vi "main.vi"() -> ()   [LabVIEW 2014]
uses:
  <vilib>/Instr/_visa.llb/VISA Configure Serial Port (Instr).vi
  <vilib>/picture/3D Picture Control/Object/Create Object (name).vi
  <vilib>/picture/3D Picture Control/NI_3D Picture Control.lvlib
panel:
  out "CALIB GZ":dbl
  out "CALIB GY":dbl
  out "CALIB GX":dbl
  out "RAW GZ":string
  out "RAW GY":string
  out "RAW GX":string
  out "ACCELEROMETER":T1(graph)
  out "AZ":string
  out "AY":string
  out "Simulator":refnum<vi>(3d-picture)
  out "CALIB GYROMETER":T1(graph)
  in  "stop":bool
  out "BYTE COUNT:":dbl
  in  "COM Port":refnum<visa-resource-name>
  out "AX":string
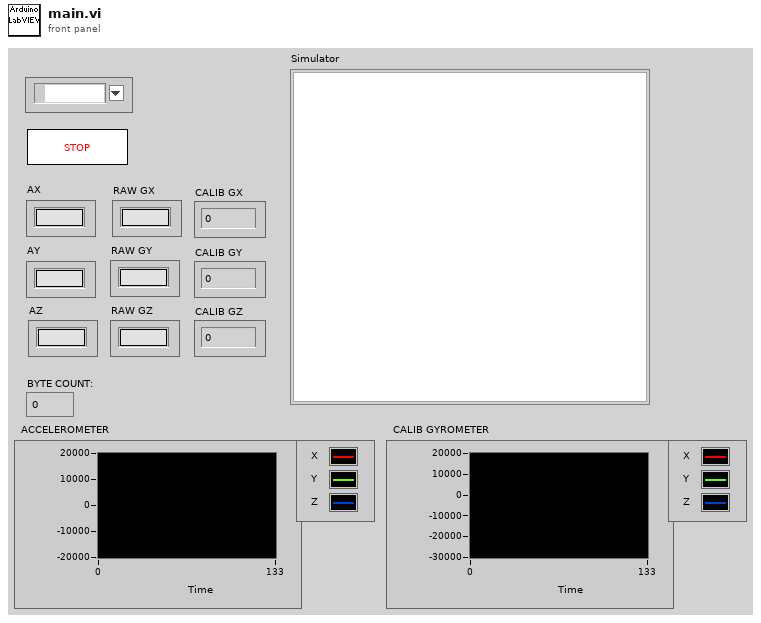
[diagram p1: front panel]
types:
  T1 = cluster{"read buffer":i32, "trimmed string":i32, "trimmed string":i32}
  T2 = enum16{"As a Decal", "With Modulation", "With Blending", "As a replacement"}
  T3 = cluster{"Red":sgl, "Green":sgl, "Blue":sgl, "Alpha":sgl}
  T4 = typedef "imagedata.ctl" = cluster{"image type":i32, "image depth":i32, "image":u8[], "mask":u8[], "colors":u32[], "Rectangle":cluster{"left":i16, "top":i16, "right":i16, "bottom":i16}}
  T5 = cluster{"trimmed string":string, "trimmed string":string, "trimmed string":string}
  T6 = cluster{"trimmed string":i32, "trimmed string":i32, "trimmed string":i32}
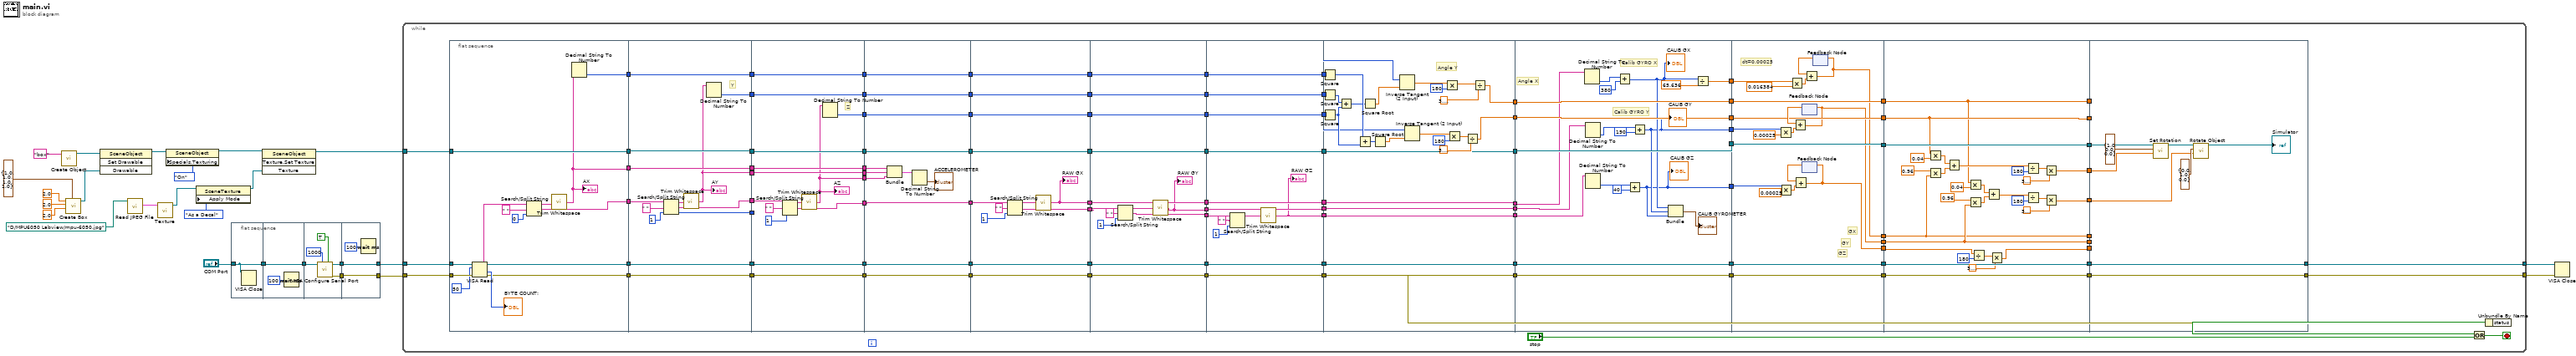
[diagram p0: block diagram]
diagram:
  n1 = call-poly <vilib>:"Create Object.vi"("Name"="box") -> ("Scene:New Object"=w1:refnum<vi>)  [unwired: 9 in, 1 out]
  n2 = call <vilib>:"Create Box.vi"("Color"=T3 {"Red"=1.0, "Green"=1.0, "Blue"=1.0, "Alpha"=1.0}, "Length Z"=2.0, "Length Y"=2.0, "Length X"=2.0) -> ("New Box Refnum"=w12:refnum<vi>)  [unwired: 6 in, 1 out]
  n3 = invoke class="SceneObject" method="Set Drawable"(reference=w1, "Drawable"=w12) -> (reference out=w2:refnum<vi>)  [unwired: 2 in, 3 out]
  n4 = call <vilib>:"Read JPEG File.vi"("path to JPEG file"=path "D:/MPU6050 Labview/mpu-6050.jpg") -> ("image data"=w11:T4)  [unwired: 8 in, 2 out]
  n5 = call <vilib>:"Texture.vi"("Image"=w11) -> ("New Texture Refnum"=w9:refnum<vi>)  [unwired: 9 in, 1 out]
  n6 = property class="SceneObject"(reference=w2, "Specials.Texturing"=enum16{"Inherit Value", "Off", "On"}."On" ("Specials:Texturing")) -> (reference out=w4:refnum<vi>)  [unwired: 1 in, 1 out]
  n7 = property class="SceneTexture"(reference=w9, "Apply Mode"=T2."As a Decal") -> (reference out=w10:refnum<vi>)  [unwired: 1 in, 1 out]
  n8 = flat-sequence {
    tunnel: "COM Port" -> [w26]
    tunnel: [w26] -> w25
    tunnel: w25 -> [w28]
    tunnel: [w28] -> w24
    tunnel: w24 -> [w33]
    tunnel: [w32] -> w23
    tunnel: [w31] -> w22
    tunnel: [w35] -> w19
    tunnel: [w36] -> w20
    tunnel: w23 -> [w36]
    tunnel: w22 -> [w35]
    frame #0 {
      n9 = VISA Close(VISA resource name=w26) -> ()  [unwired: 1 in, 1 out]
    }
    frame #1 {
      n10 = Wait (ms)(milliseconds to wait=u32 100) -> ()  [unwired: 1 out]
    }
    frame #2 {
      n11 = call-poly "VISA Configure Serial Port"("VISA resource name"=w33, "timeout (10sec)"=u32 1000, "Enable Termination\nChar (T)"=TRUE ("Enable Termination\nChar (T)")) -> ("VISA resource name out"=w32:refnum<visa-resource-name>, "error out"=w31:errorcluster)  [unwired: 11 in]
    }
    frame #3 {
      n12 = Wait (ms)(milliseconds to wait=u32 100) -> ()  [unwired: 1 out]
    }
  }
  n13 = invoke class="SceneObject" method="Texture.Set Texture"(reference=w4, "Texture"=w10) -> (reference out=w7:refnum<vi>)  [unwired: 2 in, 3 out]
  n14 = while {
    tunnel: w20 -> [w136]
    tunnel: w19 -> [w135]
    tunnel: [w131] -> w17
    tunnel: [w130] -> w18
    tunnel: w7 -> [w127]
    stop <- w132 stop-if-true
    n15 = flat-sequence {
      tunnel: w136 -> [w150]
      tunnel: w135 -> [w149]
      tunnel: [w145] -> w98
      tunnel: [w144] -> w97
      tunnel: [w143] -> w96
      tunnel: w127 -> [w143]
      tunnel: [w137] -> w95
      tunnel: [w140] -> w94
      tunnel: [w138] -> w78
      tunnel: w98 -> [w163]
      tunnel: [w163] -> w93
      tunnel: w97 -> [w162]
      tunnel: [w162] -> w92
      tunnel: w96 -> [w161]
      tunnel: [w161] -> w91
      tunnel: w95 -> [w160]
      tunnel: [w160] -> w90
      tunnel: [w157] -> w89
      tunnel: w94 -> [w159]
      tunnel: [w156] -> w88
      tunnel: [w155] -> w87
      tunnel: [w154] -> w79
      tunnel: w78 -> [w154]
      tunnel: [w152] -> w77
      tunnel: w93 -> [w177]
      tunnel: [w177] -> w86
      tunnel: w92 -> [w176]
      tunnel: [w176] -> w85
      tunnel: w91 -> [w175]
      tunnel: [w175] -> w84
      tunnel: w90 -> [w174]
      tunnel: [w174] -> w83
      tunnel: w89 -> [w173]
      tunnel: [w173] -> w82
      tunnel: [w170] -> w81
      tunnel: w88 -> [w172]
      tunnel: w87 -> [_]
      tunnel: [w169] -> w80
      tunnel: w79 -> [w169]
      tunnel: w77 -> [w168]
      tunnel: [w168] -> w76
      tunnel: [w167] -> w75
      tunnel: [w165] -> w73
      tunnel: [w189] -> w72
      tunnel: [w188] -> w71
      tunnel: [w187] -> w70
      tunnel: [w186] -> w69
      tunnel: [w185] -> w68
      tunnel: [w184] -> w67
      tunnel: w75 -> [w178]
      tunnel: w76 -> [w182]
      tunnel: w80 -> [w183]
      tunnel: w81 -> [w184]
      tunnel: w82 -> [w185]
      tunnel: w83 -> [w186]
      tunnel: w84 -> [w187]
      tunnel: w85 -> [w188]
      tunnel: w86 -> [w189]
      tunnel: w73 -> [w179]
      tunnel: [w178] -> w66
      tunnel: w72 -> [w201]
      tunnel: [w201] -> w65
      tunnel: w71 -> [w200]
      tunnel: [w200] -> w64
      tunnel: w70 -> [w199]
      tunnel: [w199] -> w63
      tunnel: w69 -> [w198]
      tunnel: [w198] -> w62
      tunnel: w68 -> [w197]
      tunnel: [w197] -> w61
      tunnel: w67 -> [w196]
      tunnel: [w196] -> w60
      tunnel: [w191] -> w59
      tunnel: [w192] -> w58
      tunnel: w66 -> [w193]
      tunnel: w65 -> [w214]
      tunnel: [w214] -> w57
      tunnel: w64 -> [w213]
      tunnel: [w213] -> w55
      tunnel: w63 -> [w212]
      tunnel: [w212] -> w53
      tunnel: w62 -> [w211]
      tunnel: [w211] -> w51
      tunnel: w61 -> [w210]
      tunnel: [w210] -> w49
      tunnel: w60 -> [w209]
      tunnel: [w209] -> w47
      tunnel: w59 -> [w205]
      tunnel: w58 -> [w206]
      tunnel: [w205] -> w45
      tunnel: [w203] -> w44
      tunnel: [w204] -> w43
      tunnel: w57 -> [w227]
      tunnel: [w227] -> w56
      tunnel: w55 -> [w226]
      tunnel: [w226] -> w54
      tunnel: w53 -> [w225]
      tunnel: [w225] -> w52
      tunnel: w51 -> [w224]
      tunnel: [w224] -> w50
      tunnel: w49 -> [w223]
      tunnel: [w223] -> w48
      tunnel: w47 -> [w222]
      tunnel: [w222] -> w46
      tunnel: w45 -> [w219]
      tunnel: w44 -> [w218]
      tunnel: w43 -> [w217]
      tunnel: [w219] -> w42
      tunnel: [w218] -> w40
      tunnel: [w216] -> w38
      tunnel: w56 -> [w253]
      tunnel: [w253] -> w126
      tunnel: w54 -> [w252]
      tunnel: [w252] -> w125
      tunnel: w52 -> [w233]
      tunnel: w50 -> [w237]
      tunnel: w48 -> [w235]
      tunnel: w46 -> [w251]
      tunnel: [w231] -> w124
      tunnel: [w232] -> w123
      tunnel: [w233] -> w100
      tunnel: [w230] -> w74
      tunnel: w42 -> [w230]
      tunnel: [w229] -> w41
      tunnel: w40 -> [w229]
      tunnel: [w228] -> w39
      tunnel: w38 -> [w228]
      tunnel: [w268] -> w129
      tunnel: [w267] -> w128
      tunnel: [w270] -> w122
      tunnel: [w256] -> w121
      tunnel: w126 -> [w268]
      tunnel: w125 -> [w267]
      tunnel: w124 -> [w271]
      tunnel: w123 -> [w272]
      tunnel: [w273] -> w120
      tunnel: [w272] -> w105
      tunnel: [w271] -> w102
      tunnel: w100 -> [w273]
      tunnel: w74 -> [w266]
      tunnel: w41 -> [w265]
      tunnel: w39 -> [w264]
      tunnel: [w254] -> w37
      tunnel: w129 -> [w293]
      tunnel: w128 -> [w292]
      tunnel: w122 -> [w276]
      tunnel: w121 -> [w286]
      tunnel: w120 -> [w281]
      tunnel: [w293] -> w109
      tunnel: [w292] -> w111
      tunnel: [w281] -> w113
      tunnel: [w278] -> w115
      tunnel: [w277] -> w117
      tunnel: [w275] -> w119
      tunnel: [w280] -> w106
      tunnel: w105 -> [w280]
      tunnel: [w279] -> w103
      tunnel: w102 -> [w279]
      tunnel: w37 -> [w274]
      tunnel: w119 -> [w298]
      tunnel: [w298] -> w118
      tunnel: w117 -> [w308]
      tunnel: [w308] -> w116
      tunnel: w115 -> [w300]
      tunnel: [w299] -> w114
      tunnel: w113 -> [w323]
      tunnel: [w323] -> w112
      tunnel: w111 -> [w322]
      tunnel: [w322] -> w110
      tunnel: w109 -> [w321]
      tunnel: [w321] -> w108
      tunnel: [w295] -> w107
      tunnel: w106 -> [w295]
      tunnel: [w297] -> w104
      tunnel: w103 -> [w297]
      tunnel: [w314] -> w101
      tunnel: [w304] -> w99
      tunnel: [w331] -> w130
      tunnel: [w332] -> w131
      tunnel: w118 -> [_]
      tunnel: w116 -> [_]
      tunnel: w114 -> [_]
      tunnel: w112 -> [w330]
      tunnel: w110 -> [w331]
      tunnel: w108 -> [w332]
      tunnel: w107 -> [_]
      tunnel: w104 -> [_]
      tunnel: w101 -> [w328]
      tunnel: w99 -> [w324]
      frame #0 {
        n16 = VISA Read(VISA resource name=w150, byte count=50, error in (no error)=w149) -> (VISA resource name out=w145:refnum<visa-resource-name>, read buffer=w142:string, return count=→"BYTE COUNT:":u32, error out=w144:errorcluster)
        n17 = Search/Split String(string=w142, search string/char (-)=" ", offset (0)=0) -> (substring before match=w139:string, match + rest of string=w140:string)  [unwired: 1 out]
        n18 = call <vilib>:"Trim Whitespace.vi"("string"=w139) -> ("trimmed string"=w138:string)  [unwired: 1 in]
        "AX" <- w138
        n19 = Decimal String To Number(string=w138) -> (number=w137:i32)  [unwired: 2 in, 1 out]
      }
      frame #1 {
        # "Y"
        n20 = Search/Split String(string=w159, search string/char (-)=" ", offset (0)=1) -> (substring before match=w153:string, match + rest of string=w156:string, offset of match=w155:i32)
        n21 = call <vilib>:"Trim Whitespace.vi"("string"=w153) -> ("trimmed string"=w152:string)  [unwired: 1 in]
        "AY" <- w152
        n22 = Decimal String To Number(string=w152) -> (number=w157:i32)  [unwired: 2 in, 1 out]
      }
      frame #2 {
        # "Z"
        n23 = Search/Split String(string=w172, search string/char (-)=" ", offset (0)=1) -> (substring before match=w166:string, match + rest of string=w167:string)  [unwired: 1 out]
        n24 = call <vilib>:"Trim Whitespace.vi"("string"=w166) -> ("trimmed string"=w165:string)  [unwired: 1 in]
        "AZ" <- w165
        n25 = Decimal String To Number(string=w165) -> (number=w170:i32)  [unwired: 2 in, 1 out]
      }
      frame #3 {
        n26 = Bundle("trimmed string"=w183, "trimmed string"=w182, "trimmed string"=w179) -> (w181:T5)  [unwired: 1 in]
        n27 = Decimal String To Number(string=w181) -> (number=→"ACCELEROMETER":T6)  [unwired: 2 in, 1 out]
      }
      frame #4 {
        n28 = Search/Split String(string=w193, search string/char (-)=" ", offset (0)=1) -> (substring before match=w194:string, match + rest of string=w192:string)  [unwired: 1 out]
        n29 = call <vilib>:"Trim Whitespace.vi"("string"=w194) -> ("trimmed string"=w191:string)  [unwired: 1 in]
        "RAW GX" <- w191
      }
      frame #5 {
        n30 = Search/Split String(string=w206, search string/char (-)=" ", offset (0)=1) -> (substring before match=w207:string, match + rest of string=w204:string)  [unwired: 1 out]
        n31 = call <vilib>:"Trim Whitespace.vi"("string"=w207) -> ("trimmed string"=w203:string)  [unwired: 1 in]
        "RAW GY" <- w203
      }
      frame #6 {
        n32 = Search/Split String(string=w217, search string/char (-)=" ", offset (0)=1) -> (substring before match=w220:string)  [unwired: 2 out]
        n33 = call <vilib>:"Trim Whitespace.vi"("string"=w220) -> ("trimmed string"=w216:string)  [unwired: 1 in]
        "RAW GZ" <- w216
      }
      frame #7 {
        # "Angle Y"
        n34 = Square(x=w237) -> (x^2=w243:i32)
        n35 = Square(x=w235) -> (x^2=w238:i32)
        n36 = Square(x=w251) -> (x^2=w250:i32)
        n37 = Add(x=w238, y=w250) -> (x+y=w242:i32)
        n38 = Add(x=w243, y=w250) -> (x+y=w239:i32)
        n39 = Square Root(x=w242) -> (sqrt(x)=w236:dbl)
        n40 = Square Root(x=w239) -> (sqrt(x)=w234:dbl)
        n41 = Inverse Tangent (2 Input)(1:w236, 2:w237) -> (0:w249:dbl)
        n42 = Inverse Tangent (2 Input)(1:w234, 2:w235) -> (0:w244:dbl)
        n43 = Multiply(x=w249, y=180) -> (x*y=w245:dbl)
        n44 = Multiply(x=w244, y=180) -> (x*y=w246:dbl)
        n45 = Divide(x=w246, y=3.141592653589793) -> (x/y=w231:dbl)
        n46 = Divide(x=w245, y=3.141592653589793) -> (x/y=w232:dbl)
      }
      frame #8 {
        # "Calib GYRO Y"
        # "Calib GYRO X"
        # "Angle X"
        n47 = Decimal String To Number(string=w266) -> (number=w263:i32)  [unwired: 2 in, 1 out]
        n48 = Decimal String To Number(string=w265) -> (number=w260:i32)  [unwired: 2 in, 1 out]
        n49 = Decimal String To Number(string=w264) -> (number=w258:i32)  [unwired: 2 in, 1 out]
        n50 = Add(x=w263, y=380) -> (x+y=w257:i32)
        "CALIB GX" <- w257
        n51 = Add(x=w258, y=40) -> (x+y=w254:i32)
        "CALIB GZ" <- w254
        n52 = Add(x=w260, y=190) -> (x+y=w256:i32)
        "CALIB GY" <- w256
        n53 = Bundle(w257, w256, w254) -> (→"CALIB GYROMETER":cluster{i32, i32, i32})  [unwired: 1 in]
        n54 = Divide(x=w257, y=65.636) -> (x/y=w270:dbl)
      }
      frame #9 {
        # "dt=0.00025"
        # "GX"
        # "GY"
        # "GZ"
        n55 = Multiply(x=w286, y=0.00025) -> (x*y=w287:dbl)
        n56 = Multiply(x=w274, y=0.00025) -> (x*y=w283:dbl)
        n57 = Multiply(x=w276, y=0.016384) -> (x*y=w290:dbl)
        n58 = feedback #1() -> (w285:dbl)  [unwired: 1 in]
        n59 = Add(x=w285, y=w287) -> (x+y=w277:dbl)
        n60 = feedback-in #1(w277) -> ()
        n61 = feedback #2() -> (w282:dbl)  [unwired: 1 in]
        n62 = Add(x=w282, y=w283) -> (x+y=w278:dbl)
        n63 = feedback-in #2(w278) -> ()
        n64 = feedback #3() -> (w289:dbl)  [unwired: 1 in]
        n65 = Add(x=w289, y=w290) -> (x+y=w275:dbl)
        n66 = feedback-in #3(w275) -> ()
      }
      frame #10 {
        n67 = Multiply(x=w297, y=0.04) -> (x*y=w318:dbl)
        n68 = Multiply(x=0.96, y=w298) -> (x*y=w317:dbl)
        n69 = Add(x=w318, y=w317) -> (x+y=w296:dbl)
        n70 = Multiply(x=w295, y=0.04) -> (x*y=w310:dbl)
        n71 = Multiply(x=0.96, y=w308) -> (x*y=w309:dbl)
        n72 = Divide(x=w300, y=180) -> (x/y=w302:dbl)
        n73 = Add(x=w310, y=w309) -> (x+y=w294:dbl)
        n74 = Multiply(x=w302, y=3.141592653589793) -> (x*y=w299:dbl)
        n75 = Divide(x=w296, y=180) -> (x/y=w315:dbl)
        n76 = Divide(x=w294, y=180) -> (x/y=w306:dbl)
        n77 = Multiply(x=w315, y=3.141592653589793) -> (x*y=w314:dbl)
        n78 = Multiply(x=w306, y=3.141592653589793) -> (x*y=w304:dbl)
      }
      frame #11 {
        n79 = call <vilib>:"Set Rotation.vi"("Angle"=w328, "Axis"=cluster{"X":sgl, "Y":sgl, "Z":sgl} {"X"=1.0, "Y"=0.0, "Z"=0.0}, "Scene Object"=w330) -> ("Rotated Scene Object"=w327:refnum<vi>)  [unwired: 7 in, 1 out]
        n80 = call <vilib>:"Rotate Object.vi"("Angle"=w324, "Axis"=cluster{"X":sgl, "Y":sgl, "Z":sgl} {"X"=0.0, "Y"=1.0, "Z"=0.0}, "Scene.Object In"=w327) -> ("Scene.Object Out"=→"Simulator":refnum<vi>)  [unwired: 7 in, 1 out]
      }
    }
    n81 = Unbundle By Name(w130) -> ("status"=w134:bool)
    n82 = Or(x=w134, y="stop") -> (x .or. y?=w132:bool)
  }
  n83 = VISA Close(VISA resource name=w17, error in (no error)=w18) -> ()  [unwired: 1 out]
